vi "Variable Drive Arm.vi"(1 "Max Speed":dbl, 2 "Wanted Angle":dbl, 3 "Encoder":dbl) -> (0 "Motor Controller":dbl)   [LabVIEW 2015]
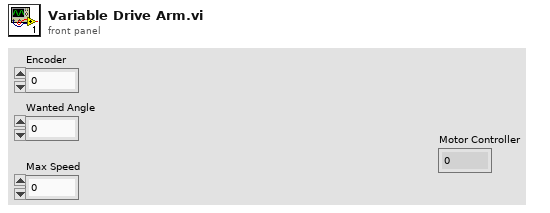
[diagram p1: front panel]
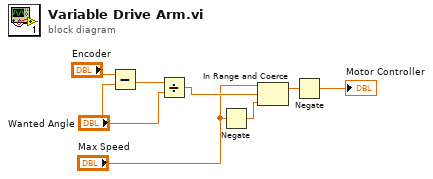
[diagram p0: block diagram]
diagram:
  n1 = Subtract(x="Encoder", y="Wanted Angle") -> (x-y=w7:dbl)
  n2 = Divide(x=w7, y="Wanted Angle") -> (x/y=w6:dbl)
  n3 = Negate(x="Max Speed") -> (-x=w5:dbl)
  n4 = In Range and Coerce(upper limit="Max Speed", x=w6, lower limit=w5) -> (coerced(x)=w2:dbl)  [unwired: 1 out]
  n5 = Negate(x=w2) -> (-x=→"Motor Controller":dbl)
